vi "File_Bitstream.vi"() -> ()   [LabVIEW 2019]
uses:
  <vilib>/addons/Modulation/niDMT.lvlib
panel:
  out "data":i8[](array[numeric])
  in  "file path (use dialog)":path
  out "Out Bitstream":i8[](array[numeric])
  in  "Packet Size":i32
  in  "Transmit":bool
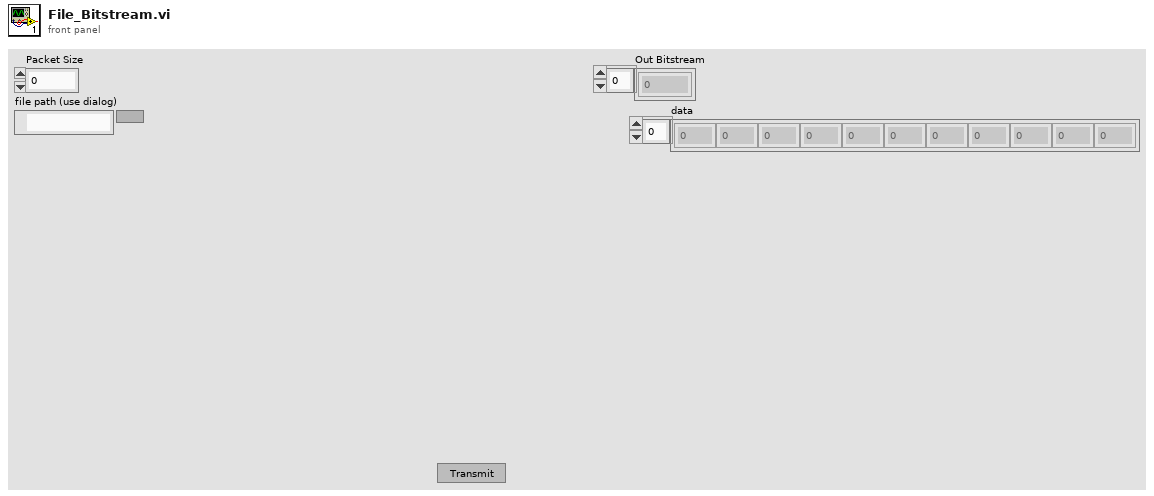
[diagram p1: front panel]
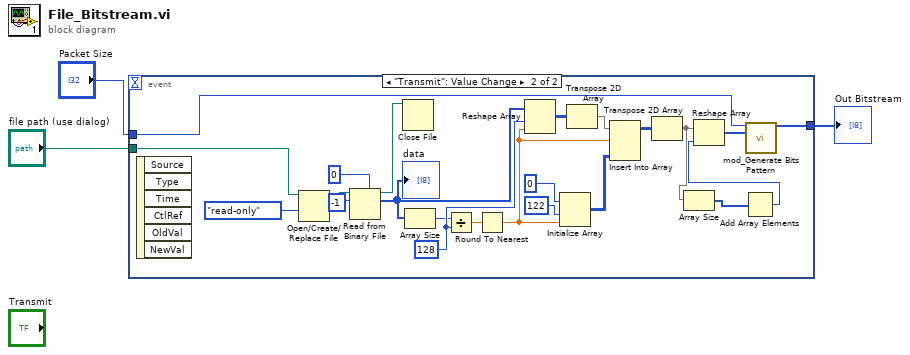
[diagram p0: block diagram]
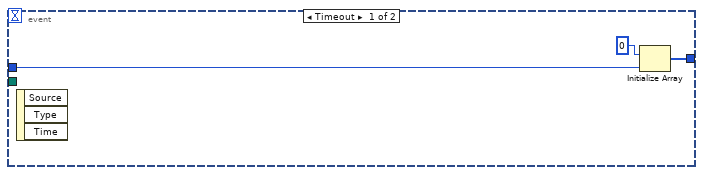
[diagram p2: hidden frame]
diagram:
  n1 = event shown="[1] \"Transmit\": Value Change" {
    selector: _ -> [_ _]
    dyn-events: _ -> [_ _]
    timeout: _ -> [_ _]
    tunnel: "Packet Size" -> [w5 w12]
    tunnel: [w4 w11] -> w2
    tunnel: "file path (use dialog)" -> [_ w29]
    event Timeout {
      n2 = event-data() -> ()  [unwired: 1 in, 3 out]
      n3 = Initialize Array(i8 0 ("element"), w5) -> (w4:i8[])
    }
    event "Transmit": Value Change {
      w23 = 128 ("dimension size")
      n4 = event-data() -> ()  [unwired: 1 in, 6 out]
      n5 = Open/Create/Replace File(file path (use dialog)=w29, access (0:read/write)=enum16{"read/write", "read-only", "write-only"}."read-only") -> (refnum out=w27:refnum<file>)  [unwired: 4 in, 2 out]
      n6 = Read from Binary File(5:i8 0 ("element"), 10:-1 ("count (1)"), 11:w27) -> (2:w24:i8[], 3:w25:refnum<file>)  [unwired: 3 in, 2 out]
      "data" <- w24
      n7 = Close File(refnum=w25) -> ()  [unwired: 1 in, 2 out]
      n8 = Array Size(array=w24) -> (size(s)=w22:i32)
      n9 = Divide(x=w22, y=w23) -> (x/y=w21:dbl)
      n10 = Round To Nearest(number=w21) -> (nearest integer value=w15:dbl)
      n11 = Reshape Array(w24, w23, w15) -> (w20:i8[][])
      n12 = Initialize Array(i8 0 ("element"), 122 ("dimension size"), w15) -> (w16:i8[][])
      n13 = Transpose 2D Array(2D array=w20) -> (transposed array=w17:i8[][])
      n14 = Insert Into Array(array=w17, index (row)=w15, new element=w16) -> (w14:i8[][])  [unwired: 1 in]
      n15 = Transpose 2D Array(2D array=w14) -> (transposed array=w10:i8[][])
      n16 = Array Size(array=w10) -> (size(s)=w9:i32[])
      n17 = Add Array Elements(numeric array=w9) -> (sum=w8:i32)
      n18 = Reshape Array(w10, w8) -> (w13:i8[])
      n19 = call <vilib>:"mod_Generate Bits Pattern.vi"("Total Bits"=w12, "User Base Bit Pattern"=w13) -> ("Output Bit Stream"=w11:i8[])  [unwired: 13 in]
    }
  }
  "Out Bitstream" <- w2
